vi "NewtonsPSM_Range.vi"(0 "VISA session":refnum<visa-resource-name>, 1 "Input Connection (Main)":u16(ring) items=["MAIN", "SECONDARY", "DIFFERENTIAL"], 2 "Input Coupling (Internal)":u16(ring) items=["AC+DC", "AC"], 5 "Input Ranging Mode (Auto)":u16(ring) items=["AUTO", "UPAUTO", "1mV", "3mV", "10mV", "30mV", "100mV", "300mV", "1V", "3V", "10V"], 7 "Input Input Type (Internal)":u16(ring)=1 items=["DISABLED", "INTERNAL", "EXTERNAL SHUNT"], 9 "Input Voltage Scale factor (1)":dbl=1.0 min=0.0 max=100000.0 step=0.001, 11 "error in (no error)":errorcluster, 12 "Input Shunt Value (0,02)":dbl=0.02 min=1e-06 max=10.0 step=1e-06, 13 "Input Selection (CH1)":u16(ring) items=["CH1", "CH2"]) -> (4 "dup VISA session":refnum<visa-resource-name>, 15 "error out":errorcluster)   [LabVIEW 2025, in "NewtonsPSM1735.lvlib"]
doc: "This VI set the ranging parameters for voltage and current of the PPA2530"
uses:
  NewtonsPSM1735.lvlib
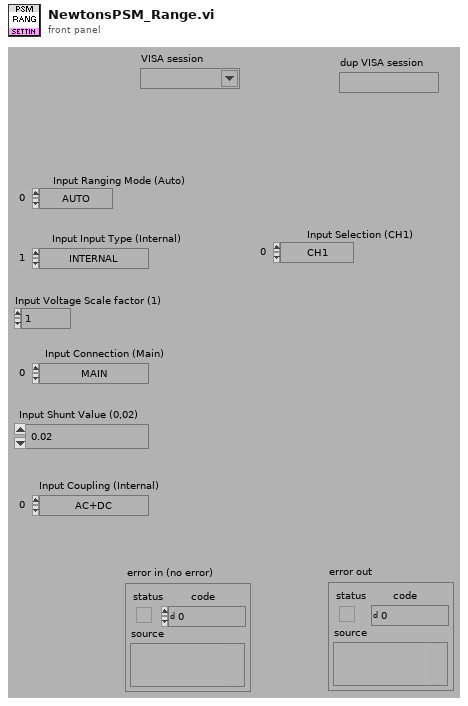
[diagram p1: front panel]
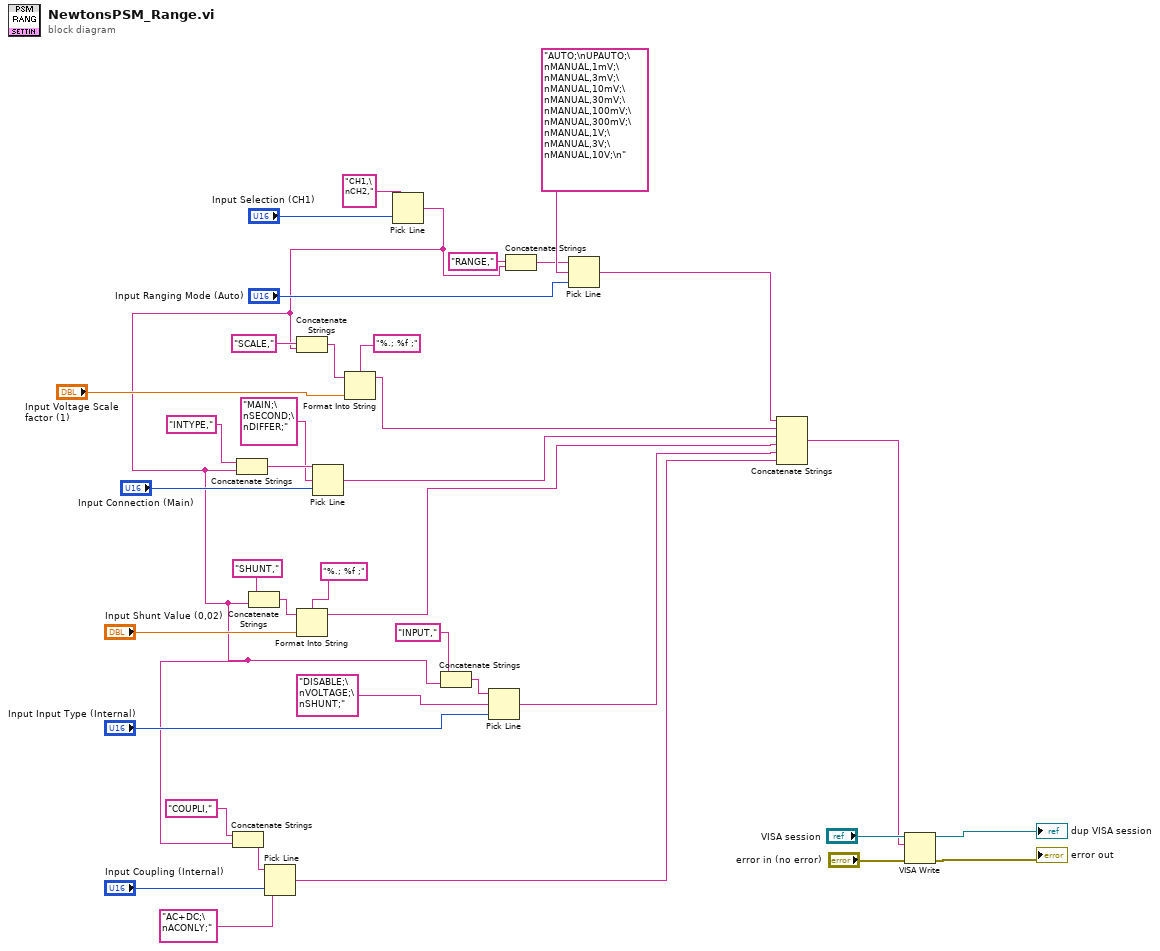
[diagram p0: block diagram]
diagram:
  n1 = Pick Line(multi-line string="CH1,\nCH2," ("chaîne multiligne"), line index="Input Selection (CH1)") -> (output string=w10:string)  [unwired: 1 out]
  n2 = Concatenate Strings("COUPLI," ("chaîne"), w10) -> (w11:string)
  n3 = Concatenate Strings("INTYPE," ("chaîne multiligne"), w10) -> (w24:string)
  n4 = Concatenate Strings("SHUNT," ("chaîne"), w10) -> (w19:string)
  n5 = Pick Line(string ("")=w11, multi-line string="AC+DC;\nACONLY;" ("chaîne multiligne"), line index="Input Coupling (Internal)") -> (output string=w1:string)
  n6 = Concatenate Strings("SCALE,", w10) -> (w25:string)
  n7 = Format Into String(format string="%.; %f ;" ("chaîne de format"), initial string=w19, "Input Shunt Value (0,02)") -> (resulting string=w3:string)  [unwired: 1 in, 1 out]
  n8 = Pick Line(string ("")=w24, multi-line string="MAIN;\nSECOND;\nDIFFER;" ("chaîne multiligne"), line index="Input Connection (Main)") -> (output string=w4:string)
  n9 = Format Into String(format string="%.; %f ;" ("chaîne de format"), initial string=w25, "Input Voltage Scale factor (1)") -> (resulting string=w5:string)  [unwired: 1 in, 1 out]
  n10 = Concatenate Strings("INPUT,", w10) -> (w15:string)
  n11 = Pick Line(string ("")=w15, multi-line string="DISABLE;\nVOLTAGE;\nSHUNT;", line index="Input Input Type (Internal)") -> (output string=w2:string)
  n12 = Concatenate Strings("RANGE,", w10) -> (w27:string)
  n13 = Pick Line(string ("")=w27, multi-line string="AUTO;\nUPAUTO;\nMANUAL,1mV;\nMANUAL,3mV;\nMANUAL,10mV;\nMANUAL,30mV;\nMANUAL,100mV;\nMANUAL,300mV;\nMANUAL,1V;\nMANUAL,3V;\nMANUAL,10V;\n", line index="Input Ranging Mode (Auto)") -> (output string=w6:string)
  n14 = Concatenate Strings(w6, w5, w4, w3, w2, w1) -> (w7:string)
  n15 = VISA Write(VISA resource name="VISA session", write buffer=w7, error in (no error)="error in (no error)") -> (VISA resource name out=→"dup VISA session":refnum<visa-resource-name>, error out=→"error out":errorcluster)  [unwired: 1 out]
